vi "04_QControl_AdjMCLB.vi"() -> ()   [LabVIEW 2020]
uses:
  AdjMCLB/AdjMCLB.lvclass
  a1c3afd6-ccd7-4a4c-8690-1d5eaf0ffe36.vi
  5f76a05e-377a-4760-9f1e-ec6ff57fe28f.vi
panel:
  in  "Multicolumn Listbox":i32(listbox)
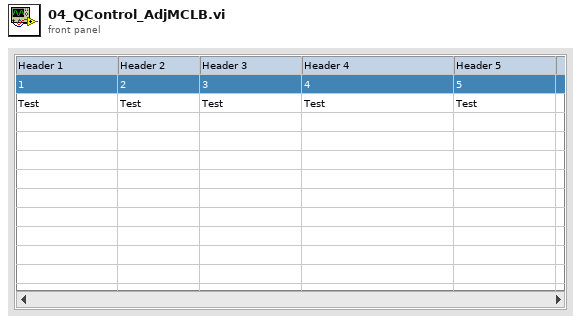
[diagram p1: front panel]
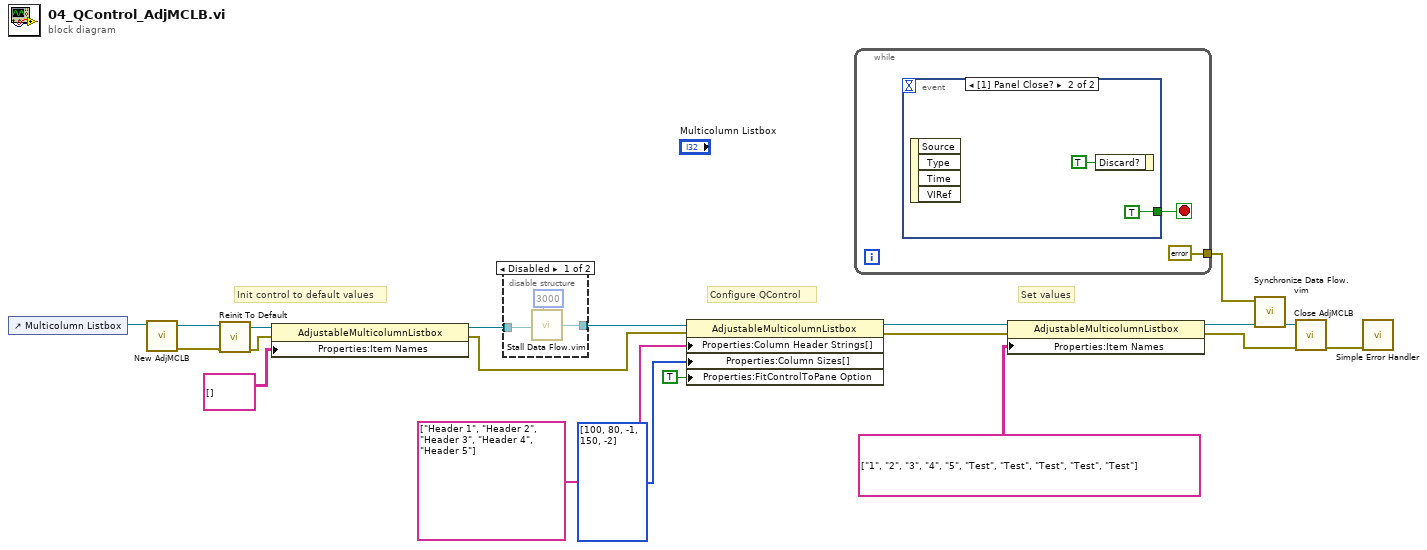
[diagram p0: block diagram]
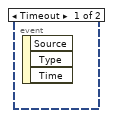
[diagram p2: hidden frame]
diagram:
  # "Set values"
  # "Configure QControl"
  # "Init control to default values"
  n1 = control-ref of="Multicolumn Listbox"() -> (w20:refnum<vi>)
  n2 = call "New AdjMCLB.vi"("Reference"=w20) -> ("error out"=w7:errorcluster, "AdjustableMulticolumnListbox out"=w8:refnum<class "AdjMCLB.lvclass">)  [unwired: 9 in]
  n3 = call-dynamic "Reinit To Default.vi"("error in (no error)"=w7, "Control in"=w8) -> ("error out"=w2:errorcluster, "Control out"=w5:refnum<class "AdjMCLB.lvclass">)  [unwired: 8 in]
  n4 = property class="AdjustableMulticolumnListbox"(reference=w5, error in=w2, "Properties:Item Names"=string[][] [] ("Item Names")) -> (reference out=w4:refnum<class "AdjMCLB.lvclass">, error out=w3:errorcluster)
  n5 = disable-structure shown="Disabled" {
    disable-tunnel: [w23 w24] -> w6
    disable-tunnel: w4 -> [w21 w24]
    frame Disabled {
      n6 = call "Stall Data Flow.vim"("value in"=w21, "milliseconds to wait"=u32 3000) -> ("value out"=w23:refnum<class "AdjMCLB.lvclass">)  [unwired: 1 out]
    }
    frame Enabled {
    }
  }
  n7 = property class="AdjustableMulticolumnListbox"(reference=w6, error in=w3, "Properties:Column Header Strings[]"=string[] ["Header 1", "Header 2", "Header 3", "Header 4", "Header 5"] ("Column Header Strings[]"), "Properties:Column Sizes[]"=i32[] [100, 80, -1, 150, -2] ("Column Sizes[]"), "Properties:FitControlToPane Option"=TRUE ("FitControlToPane Option")) -> (reference out=w13:refnum<class "AdjMCLB.lvclass">, error out=w12:errorcluster)
  n8 = while {
    tunnel: [errorcluster {"status"=FALSE, "code"=0, "source"=""} ("error constant")] -> w18
    stop <- w26 stop-if-true
    n9 = event shown="[1] Panel Close?" {
      selector: _ -> [_ _]
      dyn-events: _ -> [_ _]
      timeout: _ -> [_ _]
      tunnel: [_ TRUE] -> w26
      event Timeout {
        n10 = event-data() -> ()  [unwired: 1 in, 3 out]
      }
      event Panel Close? {
        n11 = event-data() -> ()  [unwired: 1 in, 4 out]
        n12 = event-data("Discard?"=TRUE) -> ()  [unwired: 1 in, 1 out]
      }
    }
  }
  n13 = property class="AdjustableMulticolumnListbox"(reference=w13, error in=w12, "Properties:Item Names"=string[][] [["1", "2", "3", "4", "5"], ["Test", "Test", "Test", "Test", "Test"]] ("Item Names")) -> (reference out=w11:refnum<class "AdjMCLB.lvclass">, error out=w10:errorcluster)
  n14 = call "Synchronize Data Flow.vim"("input 4"=w11, "input 1"=w18) -> ("output 4"=w19:refnum<class "AdjMCLB.lvclass">)  [unwired: 2 in, 3 out]
  n15 = call "Close AdjMCLB.vi"("error in (no error)"=w10, "AdjustableMulticolumnListbox in"=w19) -> ("error out"=w17:errorcluster)  [unwired: 9 in]
  n16 = call <vilib>:"Simple Error Handler.vi"("error in (no error)"=w17) -> ()  [unwired: 4 in, 5 out]
